vi "MoveZContact.vi"(8 "error in (no error) 2":errorcluster, 11 "connection ID 2":refnum<k5>) -> (0 "error out":errorcluster, 3 "connection ID":refnum<k5>)   [LabVIEW 2018]
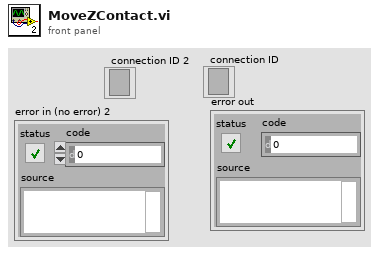
[diagram p1: front panel]
types:
  T1 = enum16{"Standard", "Buffered", "CRLF", "Immediate"}
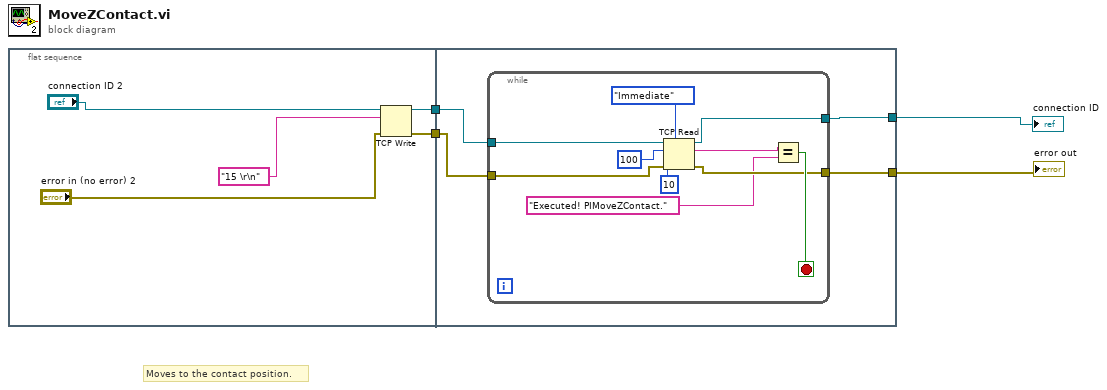
[diagram p0: block diagram]
diagram:
  # "Moves to the contact position."
  n1 = flat-sequence {
    tunnel: [w9] -> w4
    tunnel: [w8] -> w3
    tunnel: w4 -> [w12]
    tunnel: w3 -> [w13]
    tunnel: [w11] -> w2
    tunnel: [w10] -> w1
    frame #0 {
      n2 = TCP Write(connection ID="connection ID 2", data in="15 \r\n" ("format string"), error in (no error)="error in (no error) 2") -> (connection ID out=w9:refnum<k5>, error out=w8:errorcluster)  [unwired: 1 in, 1 out]
    }
    frame #1 {
      n3 = while {
        tunnel: w13 -> [w21]
        tunnel: [w17] -> w10
        tunnel: [w16] -> w11
        tunnel: w12 -> [w14]
        stop <- w18 stop-if-true
        n4 = TCP Read(connection ID=w14, bytes to read=100, error in (no error)=w21, 7:T1."Immediate" ("mode (standard)"), 9:10 ("timeout ms (25000)")) -> (connection ID out=w16:refnum<k5>, data out=w19:string, error out=w17:errorcluster)
        n5 = Equal?(x=w19, y="Executed! PIMoveZContact.") -> (x = y?=w18:bool)
      }
    }
  }
  "connection ID" <- w2
  "error out" <- w1
